vi "3.vi"() -> ()   [LabVIEW 2017]
panel:
  out "波形图表":dbl[][](graph)
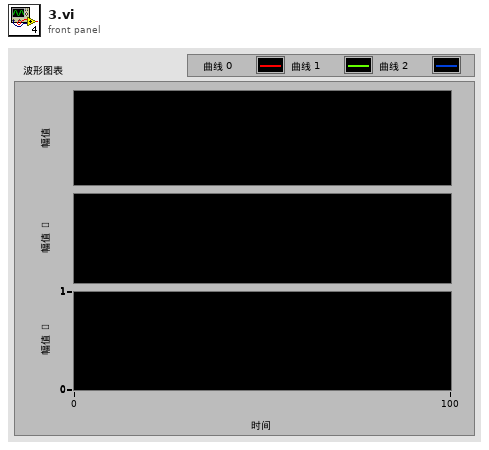
[diagram p1: front panel]
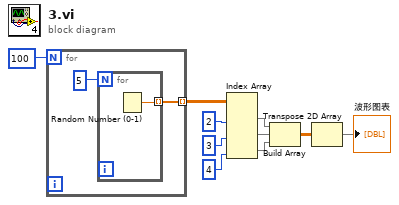
[diagram p0: block diagram]
diagram:
  n1 = for {
    N: 100 -> [_]
    tunnel: [w11] -> w9 mode=indexing
    n2 = for {
      N: 5 -> [_]
      tunnel: [w13] -> w11 mode=indexing
      n3 = Random Number (0-1)() -> (number: 0 to 1=w13:dbl)
    }
  }
  n4 = Index Array(array=w9, index (col) #1=2 ("索引 (行)"), index (col) #2=3 ("索引 (行)"), index (col) #3=4 ("索引 (行)")) -> (element #1=w5:dbl[], element #2=w4:dbl[], element #3=w3:dbl[])  [unwired: 3 in]
  n5 = Build Array(w5, w4, w3) -> (w2:dbl[][])
  n6 = Transpose 2D Array(2D array=w2) -> (transposed array=→"波形图表":dbl[][])
